vi "Main Read Processed Incoming Messages.vi"(8 "error in (no error)":errorcluster, 11 "J1939 Main Configuration":T1={"Parameters"={"J1939 XNET Settings"={"XNET Database"="", "XNET Cluster"="", "CAN Port"="", "Baud rate [Bd]"=0, "Termination"=0, "Incoming Rate"=0, "Outcoming Rate"=1, "Write Decimation"=1}, "Incoming Single Point Configuraiton"={"Incoming Single Point Frame"={"ID"=[], "Conversion"=[], "Channel Array Positions"=[], "Frame Length"=[]}, "Channel Pairs"={"Chan Refs"=[], "Previous Chan Values"=[]}, "Read FIFO"=refnum}, "Outgoing Cyclic Configuraiton"={"Outgoing Cyclic Frame"={"ID"=[], "Conversion"=[], "Channel Array Positions"=[], "Frame Length"=[], "Transmit Propreties"=[]}, "Channel Pairs"={"Block Data Refs"=[], "Previous Chan Values"=[]}, "Write FIFO"=refnum}, "J1939 Monitor Settings"={"J1939 Network Address"=0, "Name"=0}, "Simulated Addresses"=[], "Simulated Addresses LUT"=variant}, "Name"="", "J1939 Cluster"={"Processed Incoming"=refnum, "Current Device Address"=0, "Processed Outgoing"=refnum, "Process Outgoing"=refnum, "Name"=0}, "References"={"BAM Buffer"=refnum, "CM Buffer"=refnum, "CM Gen"=refnum, "BAM Gen"=refnum, "Address Claims"=refnum, "RQST"=refnum}, "StopRef"=refnum, "Frame In"="", "Frame Out"="", "Incoming Timeout"=0, "Outgoing Timeout"=0, "Listener ID"=refnum, "Parent VI Ref"=refnum, "Data Ref"=refnum, "Scale Ref"=refnum, "Incoming Direct Access"={"Offset"=0, "Length"=0}, "Outgoing Direct Access"={"Offset"=0, "Length"=0}, "vi reference"=refnum, "Name and Address"="", "Simulated Addresses"=[], "Simulated Addresses LUT"=variant} {"Simulated Addresses"."Simulated Addresses"."J1939 XNET Settings"."Name" format="%.0x"; "Simulated Addresses"."Simulated Addresses"."DM1 Data"."Data Reference" format="%.0x"; "Simulated Addresses"."Simulated Addresses"."DM1 Active?"."Data Reference" format="%.0x"; "Simulated Addresses"."Simulated Addresses"."DM2 Data"."Data Reference" format="%.0x"; "Simulated Addresses"."Simulated Addresses"."DM2 Active?"."Data Reference" format="%.0x"; "Parameters"."Simulated Addresses"."Simulated Addresses"."J1939 XNET Settings"."Name" format="%.0x"; "Parameters"."J1939 Monitor Settings"."Name" format="%.0x"; "Parameters"."Outgoing Cyclic Configuraiton"."Channel Pairs"."Block Data Refs"."Data Reference" format="%.0x"; "Parameters"."Outgoing Cyclic Configuraiton"."Outgoing Cyclic Frame"."Transmit Propreties"."Transmit Time" format="%#_p"; "Parameters"."J1939 XNET Settings"."Termination" items=["Off", "On"]; "Parameters"."Incoming Single Point Configuraiton"."Channel Pairs"."Chan Refs" format="%.0x"}) -> (0 "error out":errorcluster)   [LabVIEW 2013, in "J1939 Addon Engine.lvlib"]
uses:
  J1939 Addon Engine.lvlib
  Types/Configuration Cluster.ctl
  Types/Process Parameters.ctl
  Shared/Types/XNET Settings.ctl
  Types/Incoming Single Point Configuration.ctl
  Types/Incoming Single Point Frame Pairs.ctl
  Types/Incoming Single Point Channel Pairs.ctl
  <vilib>/NI Veristand/Custom Device API/Data Reference.ctl
  Types/Outgoing Cyclic Configuration.ctl
  Types/Outgoing Cyclic Frame Pairs.ctl
  Shared/Types/XNET Frame Event Properties.ctl
  Types/Outgoing Cyclic Channel Pairs.ctl
  <vilib>/NI Veristand/Custom Device API/Block Data Reference.ctl
  Shared/Types/Monitor Settings.ctl
  Types/Simulated Settings.ctl
  Shared/Types/Compiled Simulated Settings.ctl
  Types/DTC FIFOs.ctl
  Shared/J1939 Multi Packet Frame/Types/Setup Information Cluster.ctl
  <vilib>/xnet/xnet.llb/XNET Frame CAN.ctl
  <vilib>/xnet/xnet.llb/XNET Frame Type CAN.ctl
  Shared/J1939 Utilities/Types/CAN Outgoing Message Cluster.ctl
  Shared/J1939 Multi Packet Frame/Types/TP List References.ctl
  Shared/J1939 Multi Packet Frame/Types/BAM Buffer Connections List_Ref.ctl
  Shared/J1939 Multi Packet Frame/Types/Connection Mode Generation Connection Ref.ctl
  Shared/J1939 Multi Packet Frame/Types/BAM Generation Connections List_Ref.ctl
  Shared/J1939 Multi Packet Frame/Types/Address Table Reference.ctl
  Shared/J1939 Multi Packet Frame/Types/RQST Lookup Table Reference.ctl
  Stop FG/Stop Global Ref.ctl
  Types/Data Lookup Table Reference.ctl
  Types/Conversion Lookup Table Reference.ctl
  Shared/J1939 Multi Packet Frame/Types/RQST Comm Lookup Table_Ref.ctl
  Stop FG/Stop Global Commands.ctl
  Shared/J1939 Utilities/Common Conversions.vi
  Shared/J1939 Utilities/SubVIs/Convert CAN Arb ID to J1939 ID.vi
  Shared/J1939 Multi Packet Frame/SubVIs/RQST Lookup Table Act.vi
  <vilib>/xnet/xnet.llb/XNET Convert (Frame Raw to Signal).vi
  Stop FG/Stop FG.lvlib
  Error Handling API/Error Handling API.lvlib
  Shared/J1939 Utilities/J1939 Utilities.lvlib
  <vilib>/NI Veristand/Custom Device API/Custom Device API.lvlib
  Shared/J1939 Addon Shared.lvlib
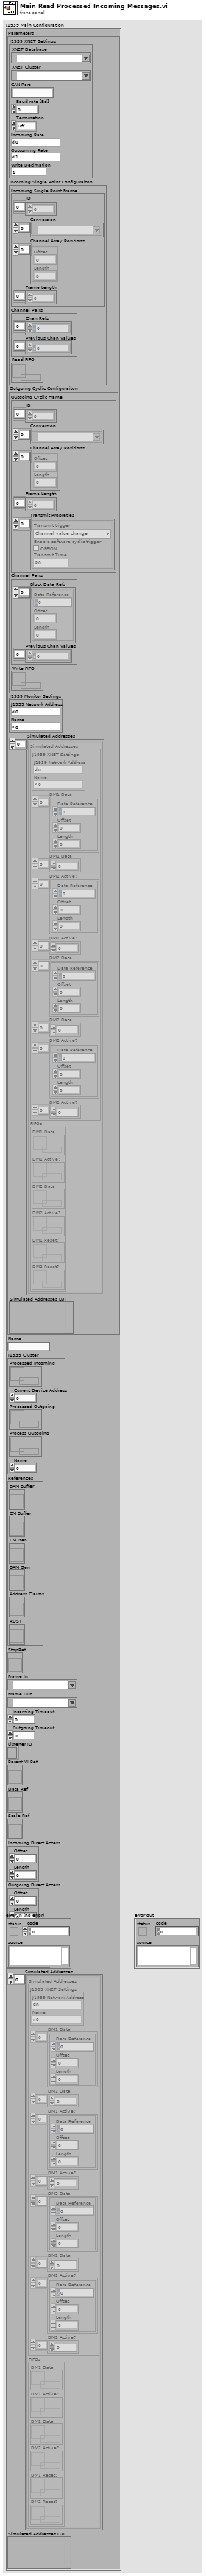
[diagram p1: front panel]
types:
  T1 = typedef "J1939 Addon Engine.lvlib/Configuration Cluster.ctl" = cluster{"Parameters":T2, "Name":string, "J1939 Cluster":T17, "References":T18, "StopRef":T24, "Frame In":refnum<k21>, "Frame Out":refnum<k21>, "Incoming Timeout":u32, "Outgoing Timeout":u32, "Listener ID":refnum<k5>, "Parent VI Ref":refnum<vi>, "Data Ref":T25, "Scale Ref":T26, "Incoming Direct Access":cluster{"Offset":u32, "Length":u32}, "Outgoing Direct Access":cluster{"Offset":u32, "Length":u32}, "vi reference":T27, "Name and Address":string, "Simulated Addresses":T14[], "Simulated Addresses LUT":variant}
  T2 = typedef "J1939 Addon Engine.lvlib/Process Parameters.ctl" = cluster{"J1939 XNET Settings":T3, "Incoming Single Point Configuraiton":T4, "Outgoing Cyclic Configuraiton":T8, "J1939 Monitor Settings":T13, "Simulated Addresses":T14[], "Simulated Addresses LUT":variant}
  T3 = typedef "J1939 Addon Shared.lvlib/XNET Settings.ctl" = cluster{"XNET Database":refnum<k21>, "XNET Cluster":refnum<k21>, "CAN Port":string, "Baud rate [Bd]":u32, "Termination":u32, "Incoming Rate":u32, "Outcoming Rate":u32, "Write Decimation":u32}
  T4 = typedef "J1939 Addon Engine.lvlib/Incoming Single Point Configuration.ctl" = cluster{"Incoming Single Point Frame":T5, "Channel Pairs":T6, "Read FIFO":refnum<k33>}
  T5 = typedef "J1939 Addon Engine.lvlib/Incoming Single Point Frame Pairs.ctl" = cluster{"ID":u32[], "Conversion":refnum<k21>[], "Channel Array Positions":cluster{"Offset":u32, "Length":u32}[], "Frame Length":u32[]}
  T6 = typedef "J1939 Addon Engine.lvlib/Incoming Single Point Channel Pairs.ctl" = cluster{"Chan Refs":T7[], "Previous Chan Values":dbl[]}
  T7 = typedef "Custom Device API.lvlib/Data Reference.ctl" = i32
  T8 = typedef "J1939 Addon Engine.lvlib/Outgoing Cyclic Configuration.ctl" = cluster{"Outgoing Cyclic Frame":T9, "Channel Pairs":T11, "Write FIFO":refnum<k33>}
  T9 = typedef "J1939 Addon Engine.lvlib/Outgoing Cyclic Frame Pairs.ctl" = cluster{"ID":u32[], "Conversion":refnum<k21>[], "Channel Array Positions":cluster{"Offset":u32, "Length":u32}[], "Frame Length":u32[], "Transmit Propreties":T10[]}
  T10 = typedef "J1939 Addon Shared.lvlib/XNET Frame Event Properties.ctl" = cluster{"Transmit trigger":enum16{"Channel value change"}, "Enable software cyclic trigger":bool, "Transmit Time":dbl}
  T11 = typedef "J1939 Addon Engine.lvlib/Outgoing Cyclic Channel Pairs.ctl" = cluster{"Block Data Refs":T12[], "Previous Chan Values":dbl[]}
  T12 = typedef "Custom Device API.lvlib/Block Data Reference.ctl" = cluster{"Data Reference":T7, "Offset":i32, "Length":i32}
  T13 = typedef "J1939 Addon Shared.lvlib/Monitor Settings.ctl" = cluster{"J1939 Network Address":u8, "Name":u64}
  T14 = typedef "J1939 Addon Engine.lvlib/Simulated Settings.ctl" = cluster{"Simulated Addresses":T15, "FIFOs":T16}
  T15 = typedef "J1939 Addon Shared.lvlib/Compiled Simulated Settings.ctl" = cluster{"J1939 XNET Settings":T13, "DM1 Data":T12[], "DM1 Data":dbl[], "DM1 Active?":T12[], "DM1 Active?":dbl[], "DM2 Data":T12[], "DM2 Data":dbl[], "DM2 Active?":T12[], "DM2 Active?":dbl[]}
  T16 = typedef "J1939 Addon Engine.lvlib/DTC FIFOs.ctl" = cluster{"DM1 Data":refnum<k33>, "DM1 Active?":refnum<k33>, "DM2 Data":refnum<k33>, "DM2 Active?":refnum<k33>, "DM1 Reset?":refnum<k33>, "DM2 Reset?":refnum<k33>}
  T17 = typedef "J1939 Addon Engine.lvlib/Setup Information Cluster.ctl" = cluster{"Processed Incoming":refnum<queue>, "Current Device Address":u8, "Processed Outgoing":refnum<queue>, "Process Outgoing":refnum<queue>, "Name":u64}
  T18 = typedef "J1939 Addon Engine.lvlib/TP List References.ctl" = cluster{"BAM Buffer":T19, "CM Buffer":T19, "CM Gen":T20, "BAM Gen":T21, "Address Claims":T22, "RQST":T23}
  T19 = typedef "J1939 Addon Engine.lvlib/BAM Buffer Connections List_Ref.ctl" = refnum<vi>
  T20 = typedef "J1939 Addon Engine.lvlib/Connection Mode Generation Connection Ref.ctl" = refnum<vi>
  T21 = typedef "J1939 Addon Engine.lvlib/BAM Generation Connections List_Ref.ctl" = refnum<vi>
  T22 = typedef "J1939 Addon Engine.lvlib/Address Table Reference.ctl" = refnum<vi>
  T23 = typedef "J1939 Addon Engine.lvlib/RQST Lookup Table Reference.ctl" = refnum<vi>
  T24 = typedef "J1939 Addon Engine.lvlib/Stop FG.lvlib/Stop Global Ref.ctl" = refnum<vi>
  T25 = typedef "J1939 Addon Engine.lvlib/Data Lookup Table Reference.ctl" = refnum<vi>
  T26 = typedef "J1939 Addon Engine.lvlib/Conversion Lookup Table Reference.ctl" = refnum<vi>
  T27 = typedef "J1939 Addon Engine.lvlib/RQST Comm Lookup Table_Ref.ctl" = refnum<vi>
  T28 = typedef "J1939 Addon Engine.lvlib/Stop FG.lvlib/Stop Global Commands.ctl" = enum16{"Write", "Read", "Reset"}
  T29 = typedef "XNET Frame CAN.ctl" = cluster{"timestamp":timestamp, "payload":u8[], "identifier":u32, "type":T30, "extended?":bool, "echo?":bool}
  T30 = typedef "XNET Frame Type CAN.ctl" = u8
  T31 = typedef "J1939 Addon Engine.lvlib/Conversion Lookup Table Parameters Cluster.ctl" = cluster{"Conversion":refnum<k21>, "Array Position":cluster{"Offset":u32, "Length":u32}, "Length":u32, "Conv ID":u32}
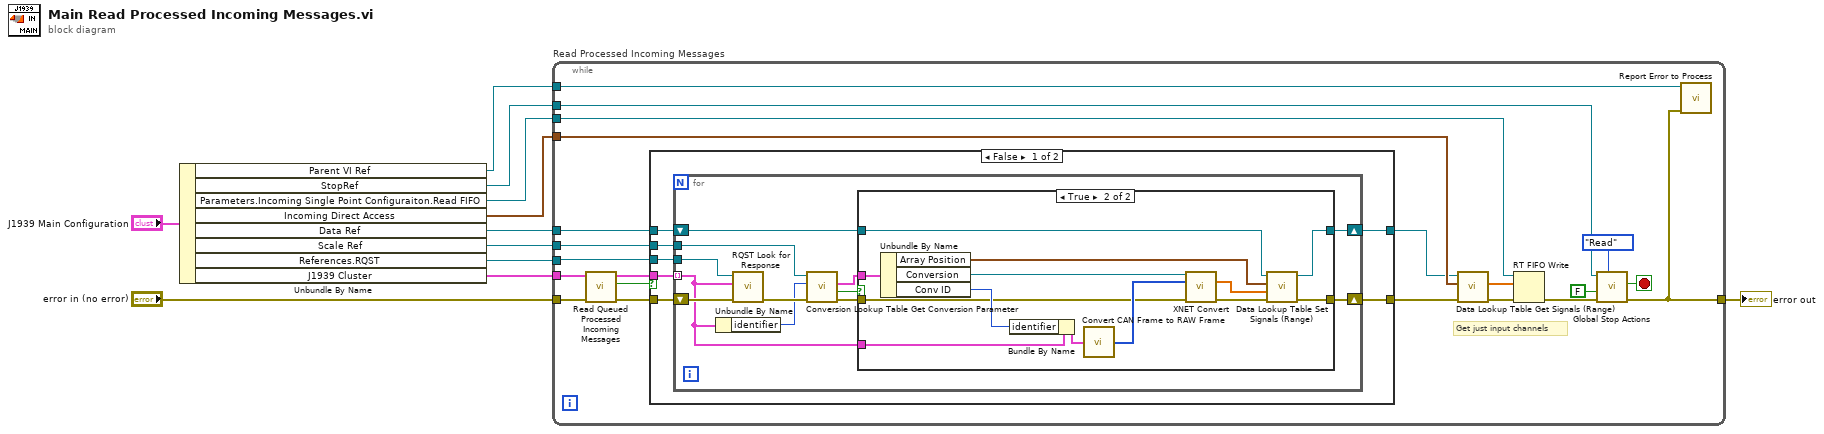
[diagram p0: block diagram]
diagram:
  n1 = Unbundle By Name("J1939 Main Configuration") -> ("Parent VI Ref"=w10:refnum<vi>, "StopRef"=w9:T24, "Parameters.Incoming Single Point Configuraiton.Read FIFO"=w8:refnum<k33>, "Incoming Direct Access"=w7:cluster{"Offset":u32, "Length":u32}, "Data Ref"=w6:T25, "Scale Ref"=w5:T26, "References.RQST"=w4:T23, "J1939 Cluster"=w11:T17)
  n2 = while "Read Processed Incoming Messages" {
    tunnel: w11 -> [w23]
    tunnel: "error in (no error)" -> [w22]
    tunnel: [w25] -> w1
    tunnel: w5 -> [w30]
    tunnel: w6 -> [w29]
    tunnel: w8 -> [w27]
    tunnel: w7 -> [w26]
    tunnel: w9 -> [w24]
    tunnel: w4 -> [w13]
    tunnel: w10 -> [w12]
    stop <- w32 stop-if-true
    # "Get just input channels"
    n3 = call "Read Queued Processed Incoming Messages.vi"("error in (no error)"=w22, "J1939 Cluster"=w23) -> ("error out"=w21:errorcluster, "timed out?"=w19:bool, "Frames"=w20:T29[])  [unwired: 7 in]
    n4 = case shown="False" w19 {
      tunnel: w30 -> [w39 _]
      tunnel: w29 -> [w38 w67]
      tunnel: [w37 w67] -> w17
      tunnel: [w36 w68] -> w16
      tunnel: w13 -> [w35 _]
      tunnel: w21 -> [w34 w68]
      tunnel: w20 -> [w33 _]
      frame False {
        n5 = for {
          tunnel: w39 -> [w51]
          tunnel: w35 -> [w47]
          shift-right: [w49] -> w37
          shift-left: w38 -> [w50]
          tunnel: w33 -> [w45] mode=indexing
          shift-right: [w48] -> w36
          shift-left: w34 -> [w46]
          n6 = Unbundle By Name(w45) -> ("identifier"=w40:u32)
          n7 = call "RQST Look for Response.vi"("error in (no error)"=w46, "CAN frame"=w45, "ref in"=w47) -> ("error out"=w41:errorcluster)  [unwired: 8 in]
          n8 = call "Conversion Lookup Table Get Conversion Parameter.vi"("error in (no error)"=w41, "ID"=w40, "Ref in"=w51) -> ("error out"=w44:errorcluster, "Found?"=w42:bool, "Parameters"=w43:T31)  [unwired: 5 in, 1 out]
          n9 = case shown="True" w42 {
            tunnel: w44 -> [w52 w55]
            tunnel: w43 -> [_ w66]
            tunnel: w50 -> [w53 w64]
            tunnel: [w52 w54] -> w48
            tunnel: [w53 w62] -> w49
            tunnel: w45 -> [_ w56]
            frame False {
            }
            frame True {
              n10 = Unbundle By Name(w66) -> ("Array Position"=w63:cluster{"Offset":u32, "Length":u32}, "Conversion"=w59:refnum<k21>, "Conv ID"=w57:u32)
              n11 = Bundle By Name(cluster=w56, "identifier"=w57) -> (w60:T29)
              n12 = call "Convert CAN Frame to RAW Frame.vi"("CAN frame"=w60) -> ("RAW Data"=w61:u8[])  [unwired: 4 in]
              n13 = call-poly <vilib>:"XNET Convert.vi"("session in"=w59, "frame data"=w61, "error in (no error)"=w55) -> ("signal data"=w58:dbl[], "error out"=w65:errorcluster)  [unwired: 10 in, 1 out]
              n14 = call "Data Lookup Table Set Signals (Range).vi"("error in (no error)"=w65, "Signals"=w58, "Direct Access"=w63, "Ref in"=w64) -> ("error out"=w54:errorcluster, "vi reference"=w62:T25)  [unwired: 6 in]
            }
          }
        }
      }
      frame True {
      }
    }
    n15 = call "Data Lookup Table Get Signals (Range).vi"("error in (no error)"=w16, "Direct Access"=w26, "Ref in"=w17) -> ("error out"=w15:errorcluster, "Signals"=w14:dbl[])  [unwired: 6 in, 1 out]
    n16 = RT FIFO Write(0:w27, 1:w14, 3:w15) -> (11:w28:errorcluster)  [unwired: 2 in, 3 out]
    n17 = call "Global Stop Actions.vi"("Command"=Stop_Global_Commands."Read", "error in (no error)"=w28, "Stop on Error?"=FALSE, "vi reference"=w24) -> ("error out"=w25:errorcluster, "Latched Stop"=w32:bool)  [unwired: 5 in, 1 out]
    n18 = call "Report Error to Process.vi"("Error"=w25, "This VI"=w12) -> ()  [unwired: 10 in]
  }
  "error out" <- w1
